vi "loadTestTime.vi"() -> ()   [LabVIEW 2012]
uses:
  <vilib>/addons/database/Connection.llb/DB Tools Open Connec (Path).vi
  <vilib>/addons/database/Connection.llb/Conn Execute.vi
  <vilib>/addons/database/Recordset.llb/Rec Destroy - Connection.vi
  <vilib>/addons/database/Recordset.llb/Rec Fetch Recordset Data (R).vi
  <vilib>/addons/database/Recordset.llb/Rec Fetch Integer Data (R).vi
  <vilib>/addons/database/_DB Variant To Data/Database Variant To Data.xnode
  <vilib>/addons/database/NI_Database_API.lvlib
panel:
  out "error out":errorcluster
  in  "Cluster":T1
  out "output cluster":T1
  out "concatenated string 3":string
  out "appended array":string[](array[string])
  out "concatenated string":string
  out "Second":dbl
  out "concatenated string 2":string
  out "TestSec":dbl
  out "Temp":i32
  out "appended array 2":i32[](array[numeric])
  out "x/y":dbl
  out "substring":string
  out "x .or. y?":bool
  out "x > y?":bool
  out "data":string
  out "error out 2":errorcluster
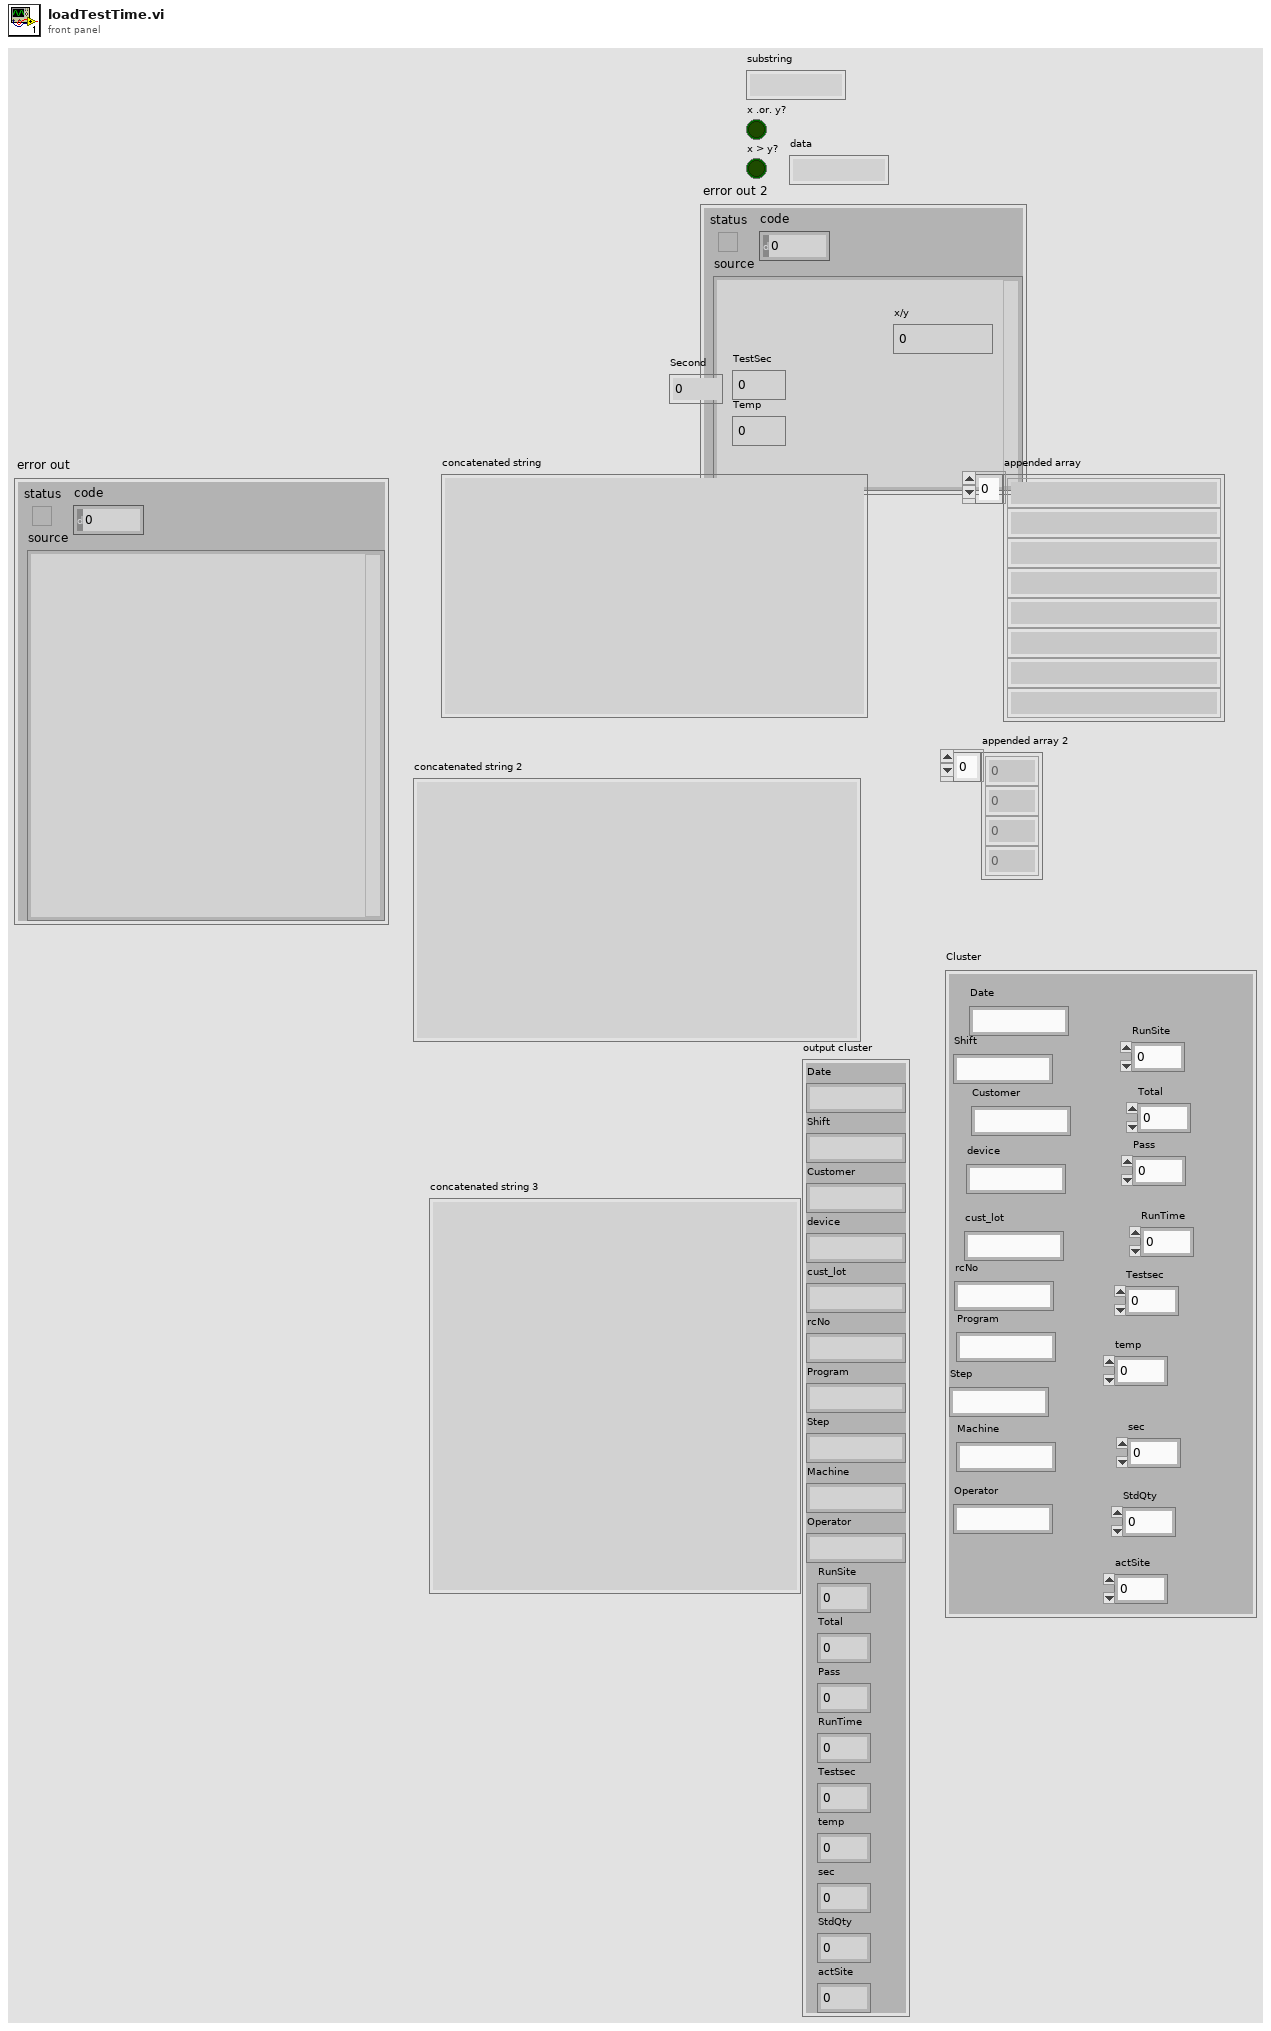
[diagram p1: front panel]
types:
  T1 = cluster{"Date":string, "Shift":string, "Customer":string, "device":string, "cust_lot":string, "rcNo":string, "Program":string, "Step":string, "Machine":string, "Operator":string, "RunSite":dbl, "Total":dbl, "Pass":dbl, "RunTime":dbl, "Testsec":dbl, "temp":dbl, "sec":dbl, "StdQty":dbl, "actSite":dbl}
  T2 = typedef "NI_Database_API.lvlib/Conn ObjectReference.ctl" = refnum<k1>
  T3 = typedef "NI_Database_API.lvlib/Rec ObjectReference.ctl" = refnum<k1>
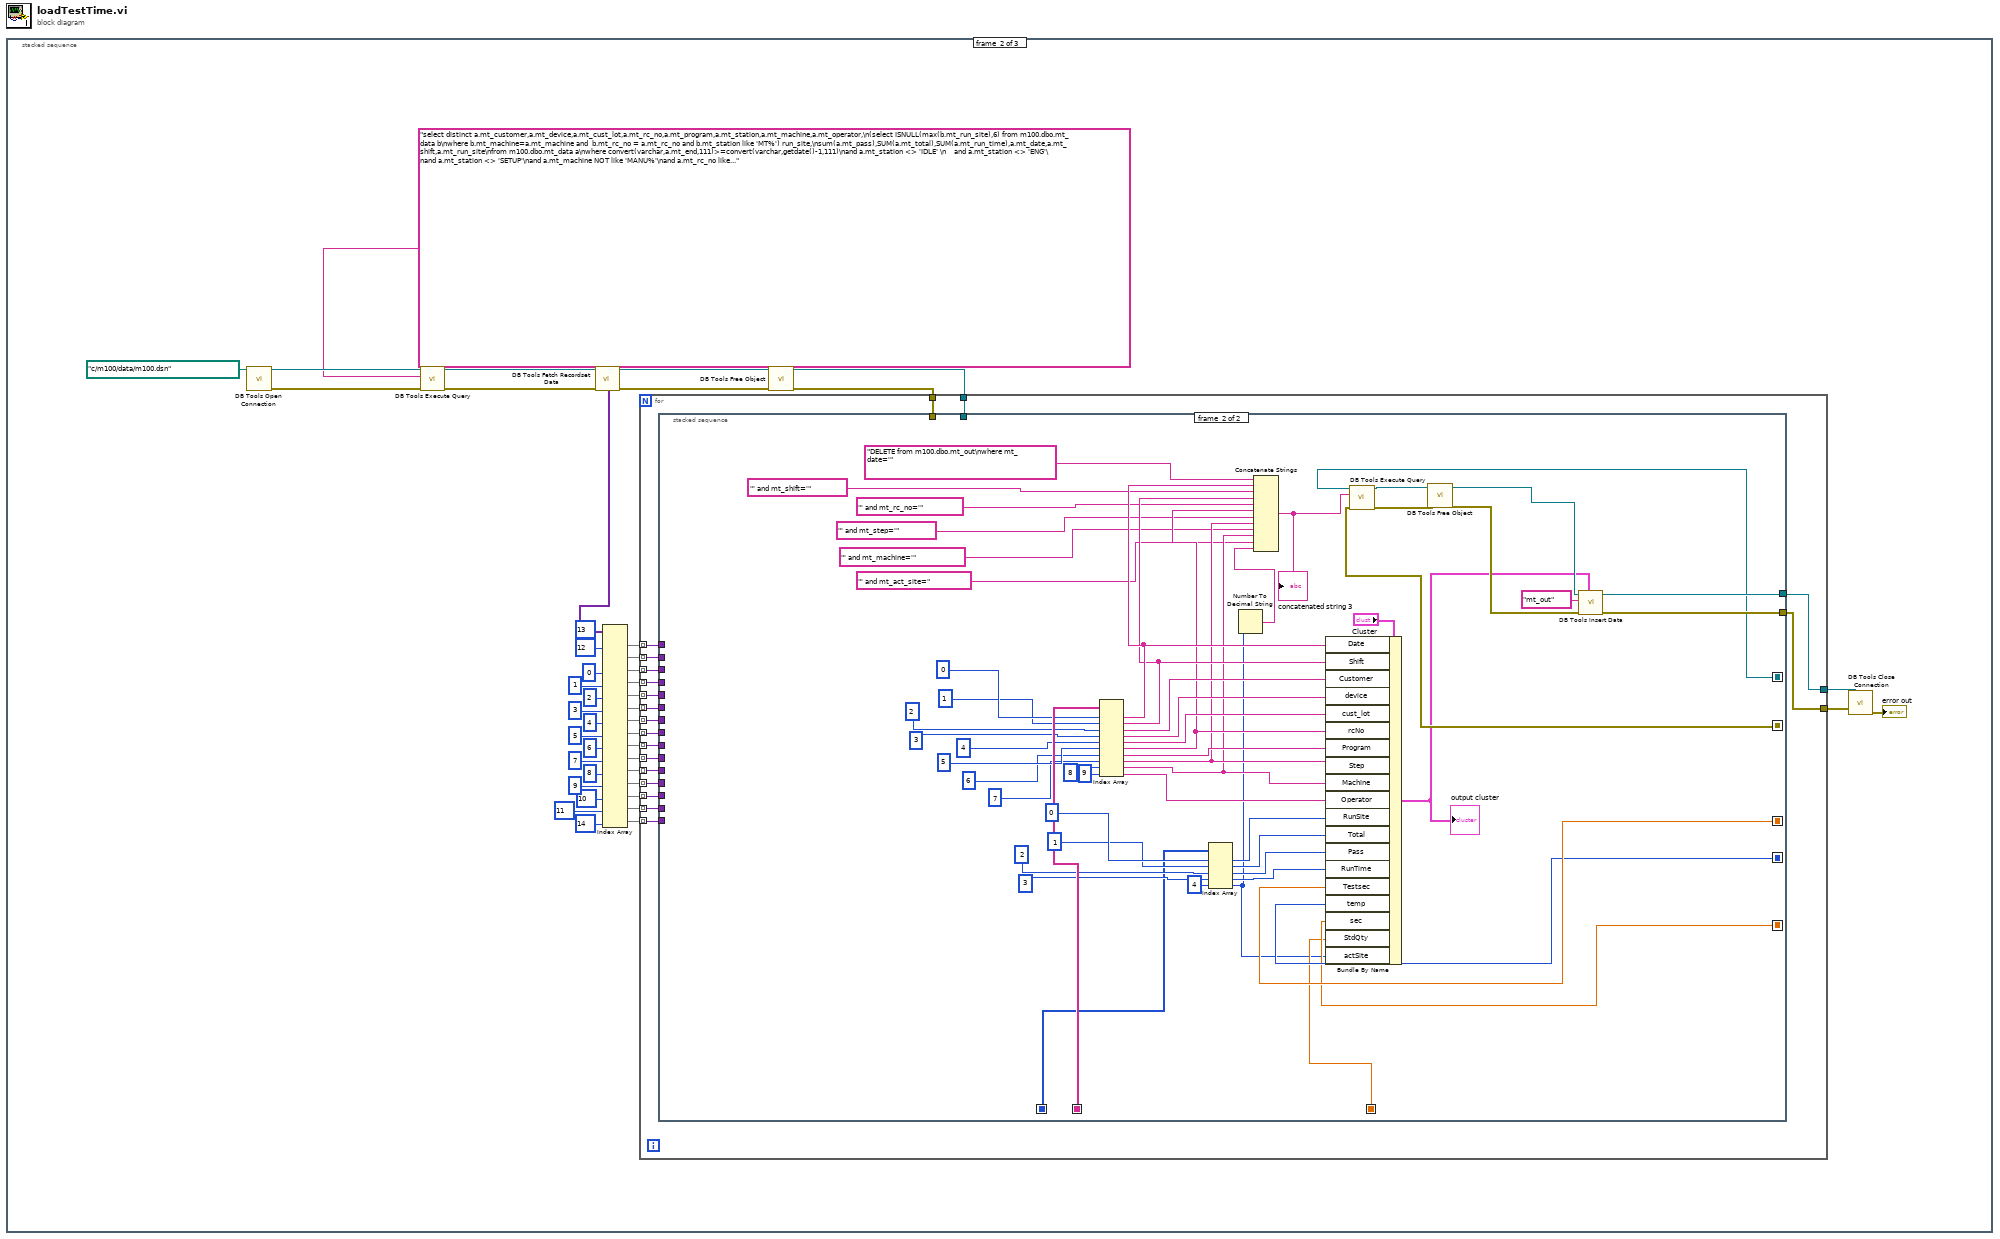
[diagram p0: block diagram]
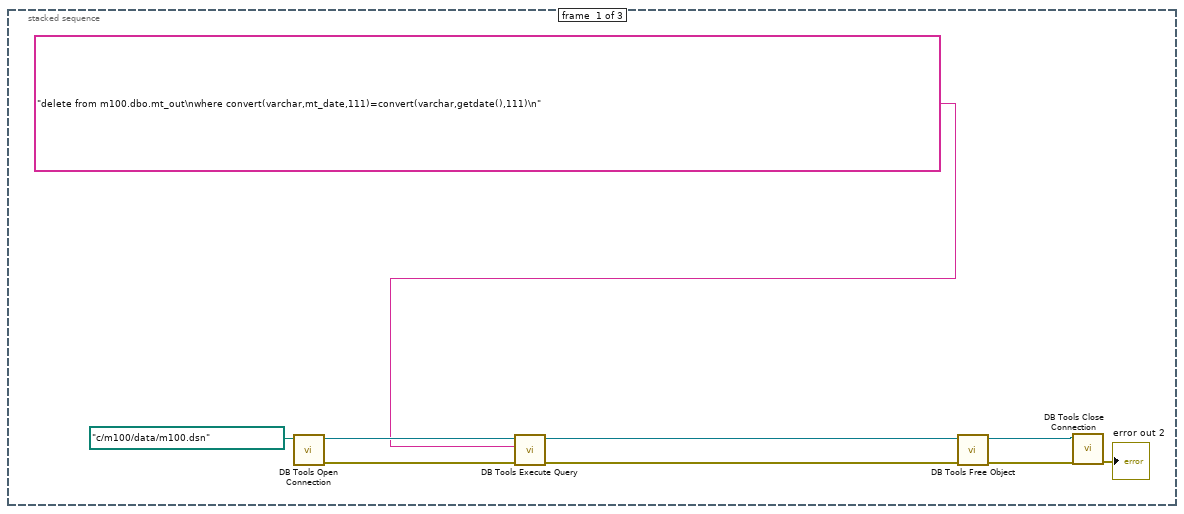
[diagram p2: hidden frame]
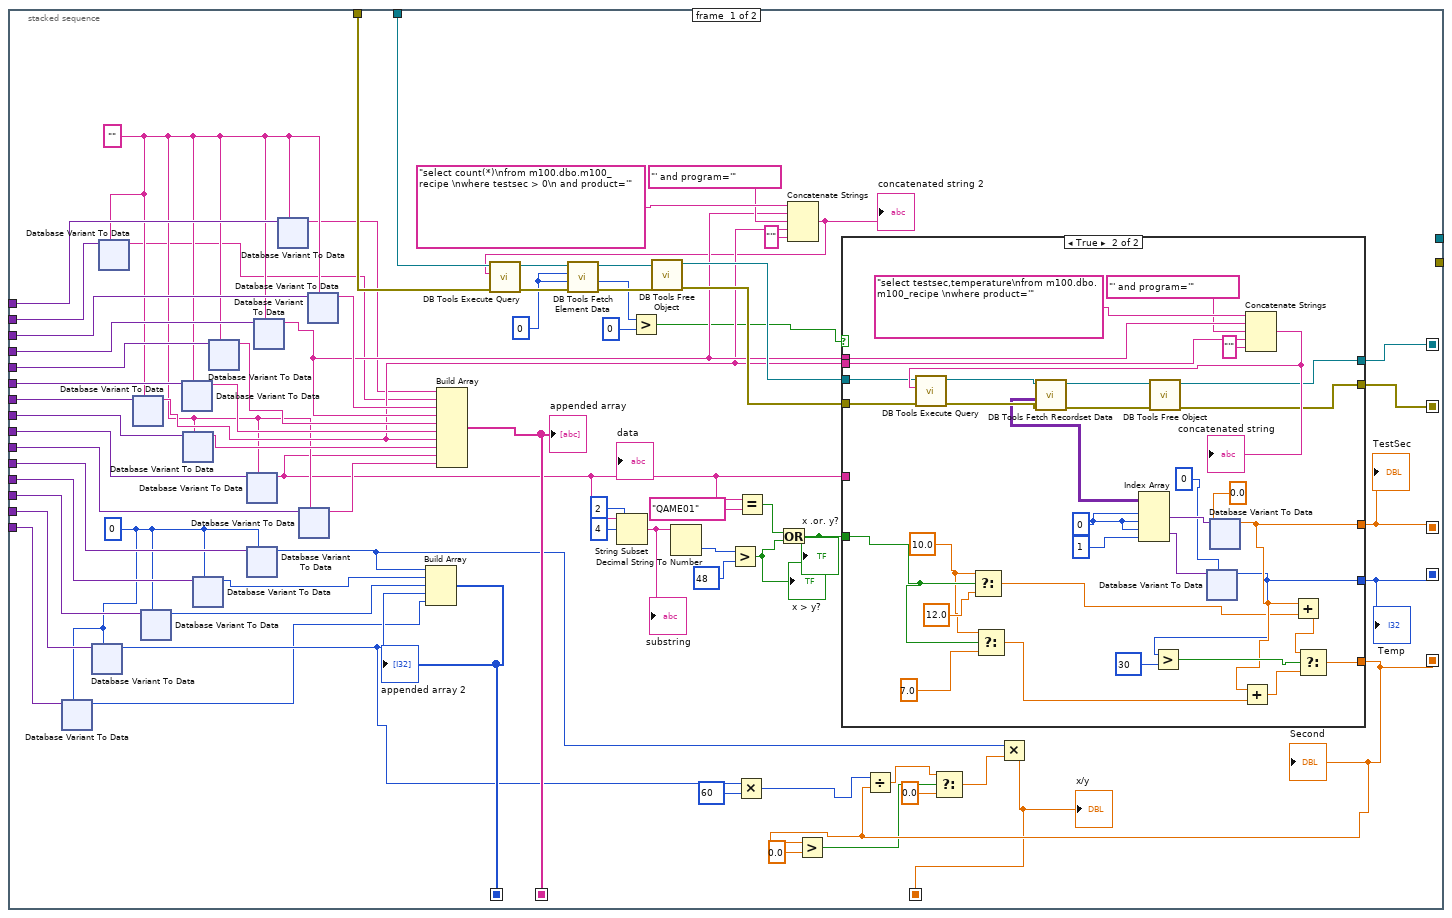
[diagram p3: hidden frame]
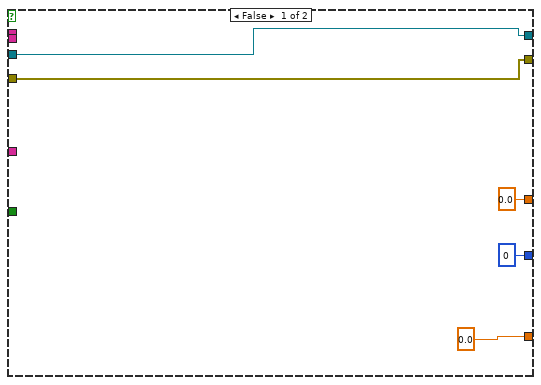
[diagram p4: hidden frame]
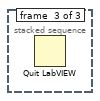
[diagram p5: hidden frame]
diagram:
  n1 = stacked-sequence {
    frame #0 {
      n2 = call-poly <vilib>:"DB Tools Open Connection.vi"("connection information"=path "c:/m100/data/m100.dsn") -> ("error out"=w8:errorcluster, "connection reference"=w9:T2)  [unwired: 7 in]
      n3 = call-poly <vilib>:"DB Tools Execute Query.vi"("error in (no error)"=w8, "SQL query"="delete from m100.dbo.mt_out\nwhere convert(varchar,mt_date,111)=convert(varchar,getdate(),111)\n", "connection reference"=w9) -> ("error out"=w4:errorcluster, "recordset reference"=w5:T3)  [unwired: 5 in]
      n4 = call-poly <vilib>:"DB Tools Free Object.vi"("error in (no error)"=w4, "recordset reference"=w5) -> ("error out"=w2:errorcluster, "connection reference"=w3:T2)  [unwired: 8 in]
      n5 = call <vilib>:"DB Tools Close Connection.vi"("error in (no error)"=w2, "connection reference"=w3) -> ("error out"=→"error out 2":errorcluster)  [unwired: 5 in]
    }
    frame #1 {
      n6 = call-poly <vilib>:"DB Tools Open Connection.vi"("connection information"=path "c:/m100/data/m100.dsn") -> ("error out"=w50:errorcluster, "connection reference"=w53:T2)  [unwired: 7 in]
      n7 = call-poly <vilib>:"DB Tools Execute Query.vi"("error in (no error)"=w50, "SQL query"="select distinct a.mt_customer,a.mt_device,a.mt_cust_lot,a.mt_rc_no,a.mt_program,a.mt_station,a.mt_machine,a.mt_operator,\n(select ISNULL(max(b.mt_run_site),6) from m100.dbo.mt_data b\nwhere b.mt_machine=a.mt_machine and  b.mt_rc_no = a.mt_rc_no and b.mt_station like 'MT%') run_site,\nsum(a.mt_pass),SUM(a.mt_total),SUM(a.mt_run_time),a.mt_date,a.mt_shift,a.mt_run_site\nfrom m100.dbo.mt_data a\nwhere convert(varchar,a.mt_end,111)>=convert(varchar,getdate()-1,111)\nand a.mt_station <> 'IDLE' \n    and a.mt_station <> 'ENG'\nand a.mt_station <> 'SETUP'\nand a.mt_machine NOT like 'MANU%'\nand a.mt_rc_no like 'A%'\ngroup by  mt_date,mt_shift,mt_customer,mt_device,mt_cust_lot,mt_rc_no,mt_program,mt_station,mt_machine,mt_operator,mt_run_site", "connection reference"=w53) -> ("error out"=w49:errorcluster, "recordset reference"=w52:T3)  [unwired: 5 in]
      n8 = call-poly <vilib>:"DB Tools Fetch Recordset Data.vi"("error in (no error)"=w49, "recordset reference"=w52) -> ("error out"=w48:errorcluster, "recordset data"=w44:variant[][], "recordset reference out"=w51:T3)  [unwired: 3 in]
      n9 = Index Array(array=w44, index (col) #1=12 ("disabled index (col)"), index (col) #2=13 ("index (col)"), index (col) #3=0 ("disabled index (col)"), index (col) #4=1 ("index (col)"), index (col) #5=2 ("index (col)"), index (col) #6=3 ("index (col)"), index (col) #7=4 ("index (col)"), index (col) #8=5 ("index (col)"), index (col) #9=6 ("index (col)"), index (col) #10=7 ("index (col)"), index (col) #11=8 ("index (col)"), index (col) #12=9 ("index (col)"), index (col) #13=10 ("index (col)"), index (col) #14=11 ("index (col)"), index (col) #15=14 ("index (col)")) -> (element #1=w13:variant[], element #2=w12:variant[], element #3=w28:variant[], element #4=w29:variant[], element #5=w30:variant[], element #6=w35:variant[], element #7=w34:variant[], element #8=w33:variant[], element #9=w32:variant[], element #10=w31:variant[], element #11=w19:variant[], element #12=w18:variant[], element #13=w17:variant[], element #14=w16:variant[], element #15=w10:variant[])  [unwired: 15 in]
      n10 = call-poly <vilib>:"DB Tools Free Object.vi"("error in (no error)"=w48, "recordset reference"=w51) -> ("error out"=w26:errorcluster, "connection reference"=w27:T2)  [unwired: 8 in]
      n11 = for {
        tunnel: w35 -> [w72] mode=indexing
        tunnel: w34 -> [w71] mode=indexing
        tunnel: w33 -> [w70] mode=indexing
        tunnel: w32 -> [w69] mode=indexing
        tunnel: w31 -> [w68] mode=indexing
        tunnel: w30 -> [w67] mode=indexing
        tunnel: w29 -> [w66] mode=indexing
        tunnel: w28 -> [w65] mode=indexing
        tunnel: w27 -> [w64]
        tunnel: w26 -> [w63]
        tunnel: [w56] -> w25
        tunnel: [w55] -> w24
        tunnel: w19 -> [w62] mode=indexing
        tunnel: w18 -> [w61] mode=indexing
        tunnel: w17 -> [w60] mode=indexing
        tunnel: w16 -> [w59] mode=indexing
        tunnel: w13 -> [w58] mode=indexing
        tunnel: w12 -> [w57] mode=indexing
        tunnel: w10 -> [w54] mode=indexing
        n12 = stacked-sequence {
          seq-local: [w106 _] -> [_ w757]
          seq-local: [w107 _] -> [_ w756]
          seq-local: [w93 _] -> [_ w755]
          seq-local: [w105 _] -> [_ w761]
          seq-local: [w104 _] -> [_ w781]
          seq-local: [w87 _] -> [_ w734]
          seq-local: [w95 _] -> [_ w738]
          seq-local: [w94 _] -> [_ w737]
          tunnel: w72 -> [w144 _]
          tunnel: w71 -> [w143 _]
          tunnel: w70 -> [w142 _]
          tunnel: w69 -> [w141 _]
          tunnel: w68 -> [w140 _]
          tunnel: w67 -> [w139 _]
          tunnel: w66 -> [w138 _]
          tunnel: w65 -> [w137 _]
          tunnel: w64 -> [w131 _]
          tunnel: w63 -> [w130 _]
          tunnel: w62 -> [w113 _]
          tunnel: w61 -> [w112 _]
          tunnel: w60 -> [w111 _]
          tunnel: w59 -> [w110 _]
          tunnel: w58 -> [w103 _]
          tunnel: w57 -> [w102 _]
          tunnel: [_ w754] -> w56
          tunnel: [_ w753] -> w55
          tunnel: w54 -> [w75 _]
          frame #0 {
            w74 = 0
            w117 = 0
            w101 = ""
            n13 = xnode "Database Variant To Data"("database variant"=w75, "type"=w74) -> ("data"=w73:i32)  [unwired: 1 in, 1 out]
            n14 = xnode "Database Variant To Data"("database variant"=w110, "type"=w74) -> ("data"=w98:i32)  [unwired: 1 in, 1 out]
            n15 = xnode "Database Variant To Data"("database variant"=w102, "type"=w101) -> ("data"=w99:string)  [unwired: 1 in, 1 out]
            n16 = xnode "Database Variant To Data"("database variant"=w143, "type"=w101) -> ("data"=w119:string)  [unwired: 1 in, 1 out]
            n17 = xnode "Database Variant To Data"("database variant"=w111, "type"=w74) -> ("data"=w108:i32)  [unwired: 1 in, 1 out]
            n18 = xnode "Database Variant To Data"("database variant"=w144, "type"=w101) -> ("data"=w134:string)  [unwired: 1 in, 1 out]
            n19 = xnode "Database Variant To Data"("database variant"=w142, "type"=w101) -> ("data"=w133:string)  [unwired: 1 in, 1 out]
            n20 = xnode "Database Variant To Data"("database variant"=w112, "type"=w74) -> ("data"=w109:i32)  [unwired: 1 in, 1 out]
            n21 = xnode "Database Variant To Data"("database variant"=w139, "type"=w101) -> ("data"=w135:string)  [unwired: 1 in, 1 out]
            n22 = xnode "Database Variant To Data"("database variant"=w141, "type"=w101) -> ("data"=w81:string)  [unwired: 1 in, 1 out]
            "data" <- w81
            n23 = xnode "Database Variant To Data"("database variant"=w113, "type"=w74) -> ("data"=w86:i32)  [unwired: 1 in, 1 out]
            n24 = xnode "Database Variant To Data"("database variant"=w138, "type"=w101) -> ("data"=w120:string)  [unwired: 1 in, 1 out]
            n25 = xnode "Database Variant To Data"("database variant"=w103, "type"=w101) -> ("data"=w100:string)  [unwired: 1 in, 1 out]
            n26 = xnode "Database Variant To Data"("database variant"=w140, "type"=w101) -> ("data"=w132:string)  [unwired: 1 in, 1 out]
            n27 = xnode "Database Variant To Data"("database variant"=w137, "type"=w101) -> ("data"=w136:string)  [unwired: 1 in, 1 out]
            n28 = Build Array(w86, w109, w108, w98, w73) -> (w105:i32[])
            "appended array 2" <- w105
            n29 = Build Array(w100, w99, w136, w120, w135, w134, w119, w133, w81, w132) -> (w104:string[])
            "appended array" <- w104
            n30 = String Subset(string=w81, offset (0)=4, length (rest)=2 ("length (rest)")) -> (substring=w84:string)
            "substring" <- w84
            n31 = Decimal String To Number(string=w84) -> (number=w83:i32)  [unwired: 2 in, 1 out]
            n32 = Greater?(x=w83, y=48) -> (0:w78:bool)
            "x > y?" <- w78
            n33 = Multiply(x=w98, y=60) -> (x*y=w96:i32)
            n34 = Equal?(x=w81, y="QAME01") -> (x = y?=w79:bool)
            n35 = Or(x=w79, y=w78) -> (x .or. y?=w77:bool)
            "x .or. y?" <- w77
            n36 = Concatenate Strings("select count(*)\nfrom m100.dbo.m100_recipe \nwhere testsec > 0\n and product='" ("SQL query"), w120, "' and program='" ("string"), w119, "'" ("string")) -> (w118:string)
            "concatenated string 2" <- w118
            n37 = call-poly <vilib>:"DB Tools Execute Query.vi"("error in (no error)"=w130, "SQL query"=w118, "connection reference"=w131) -> ("error out"=w128:errorcluster, "recordset reference"=w129:T3)  [unwired: 5 in]
            n38 = call-poly <vilib>:"DB Tools Fetch Element Data.vi"("error in (no error)"=w128, "type"=w117, "column index"=w117, "recordset reference"=w129) -> ("error out"=w126:errorcluster, "data"=w116:i32, "recordset reference out"=w127:T3)  [unwired: 3 in]
            n39 = Greater?(x=w116, y=0) -> (0:w114:bool)
            n40 = call-poly <vilib>:"DB Tools Free Object.vi"("error in (no error)"=w126, "recordset reference"=w127) -> ("error out"=w124:errorcluster, "connection reference"=w125:T2)  [unwired: 8 in]
            n41 = case shown="True" w114 {
              tunnel: w120 -> [_ w402]
              tunnel: w119 -> [_ w400]
              tunnel: w125 -> [w373 w397]
              tunnel: w124 -> [w372 w396]
              tunnel: [w373 w395] -> w95
              tunnel: [w372 w394] -> w94
              tunnel: [0.0 w382] -> w93
              tunnel: [0.0 ("data") w381] -> w106
              tunnel: [0 ("data") w380] -> w107
              tunnel: w81 -> [_ _]
              tunnel: w77 -> [_ w379]
              frame False {
              }
              frame True {
                w376 = 10.0 ("t")
                w391 = 0 ("disabled index (col)")
                n42 = Select(t=w376, s=w379, f=12.0 ("y")) -> (s? t:f=w377:dbl)
                n43 = Select(t=w376, s=w379, f=7.0 ("y")) -> (s? t:f=w374:dbl)
                n44 = Concatenate Strings("select testsec,temperature\nfrom m100.dbo.m100_recipe \nwhere product='" ("SQL query"), w402, "' and program='" ("string"), w400, "'" ("string")) -> (w399:string)
                "concatenated string" <- w399
                n45 = call-poly <vilib>:"DB Tools Execute Query.vi"("error in (no error)"=w396, "SQL query"=w399, "connection reference"=w397) -> ("error out"=w406:errorcluster, "recordset reference"=w407:T3)  [unwired: 5 in]
                n46 = call-poly <vilib>:"DB Tools Fetch Recordset Data.vi"("error in (no error)"=w406, "recordset reference"=w407) -> ("error out"=w404:errorcluster, "recordset data"=w393:variant[][], "recordset reference out"=w405:T3)  [unwired: 3 in]
                n47 = Index Array(array=w393, index (row) #1=w391, index (col) #1=w391, index (row) #2=w391, index (col) #2=1 ("index (col)")) -> (element #1=w390:variant, element #2=w389:variant)
                n48 = call-poly <vilib>:"DB Tools Free Object.vi"("error in (no error)"=w404, "recordset reference"=w405) -> ("error out"=w394:errorcluster, "connection reference"=w395:T2)  [unwired: 8 in]
                n49 = xnode "Database Variant To Data"("database variant"=w389, "type"=0) -> ("data"=w380:i32)  [unwired: 1 in, 1 out]
                n50 = Greater?(x=w380, y=30) -> (0:w385:bool)
                n51 = xnode "Database Variant To Data"("database variant"=w390, "type"=0.0) -> ("data"=w381:dbl)  [unwired: 1 in, 1 out]
                n52 = Add(x=w381, y=w374) -> (x+y=w383:dbl)
                n53 = Add(x=w381, y=w377) -> (x+y=w384:dbl)
                n54 = Select(t=w384, s=w385, f=w383) -> (s? t:f=w382:dbl)
              }
            }
            "Second" <- w93
            "TestSec" <- w106
            "Temp" <- w107
            n55 = Greater?(x=w93, y=0.0) -> (0:w90:bool)
            n56 = Divide(x=w96, y=w93) -> (x/y=w91:dbl)
            n57 = Select(t=w91, s=w90, f=0.0) -> (s? t:f=w88:dbl)
            n58 = Multiply(x=w86, y=w88) -> (x*y=w87:dbl)
            "x/y" <- w87
          }
          frame #1 {
            n59 = Index Array(array=w781, index #1=0 ("index"), index #2=1 ("index"), index #3=2 ("index"), index #4=3 ("index"), index #5=4 ("index"), index #6=5 ("index"), index #7=6 ("index"), index #8=7 ("index"), index #9=8 ("index"), index #10=9 ("index")) -> (element #1=w751:string, element #2=w749:string, element #3=w770:string, element #4=w769:string, element #5=w768:string, element #6=w747:string, element #7=w767:string, element #8=w745:string, element #9=w743:string, element #10=w766:string)
            n60 = Index Array(array=w761, index #1=0 ("index"), index #2=1 ("index"), index #3=2 ("index"), index #4=3 ("index"), index #5=4 ("index")) -> (element #1=w741:i32, element #2=w760:i32, element #3=w759:i32, element #4=w758:i32, element #5=w728:i32)
            n61 = Number To Decimal String(number=w728) -> (decimal integer string=w740:string)  [unwired: 1 in]
            n62 = Concatenate Strings("DELETE from m100.dbo.mt_out\nwhere mt_date='", w751, "' and mt_shift='" ("string"), w749, "' and mt_rc_no='" ("string"), w747, "' and mt_step='" ("string"), w745, "' and mt_machine='" ("string"), w743, "' and mt_act_site=" ("string"), w740) -> (w739:string)
            "concatenated string 3" <- w739
            n63 = Bundle By Name(cluster="Cluster", "Date"=w751, "Shift"=w749, "Customer"=w770, "device"=w769, "cust_lot"=w768, "rcNo"=w747, "Program"=w767, "Step"=w745, "Machine"=w743, "Operator"=w766, "RunSite"=w741, "Total"=w760, "Pass"=w759, "RunTime"=w758, "Testsec"=w757, "temp"=w756, "sec"=w755, "StdQty"=w734, "actSite"=w728) -> (w732:T1)
            "output cluster" <- w732
            n64 = call-poly <vilib>:"DB Tools Execute Query.vi"("error in (no error)"=w737, "SQL query"=w739, "connection reference"=w738) -> ("error out"=w729:errorcluster, "recordset reference"=w730:T3)  [unwired: 5 in]
            n65 = call-poly <vilib>:"DB Tools Free Object.vi"("error in (no error)"=w729, "recordset reference"=w730) -> ("error out"=w735:errorcluster, "connection reference"=w736:T2)  [unwired: 8 in]
            n66 = call <vilib>:"DB Tools Insert Data.vi"("data"=w732, "error in (no error)"=w735, "table"="mt_out", "connection reference"=w736) -> ("error out"=w753:errorcluster, "connection reference out"=w754:T2)  [unwired: 6 in]
          }
        }
      }
      n67 = call <vilib>:"DB Tools Close Connection.vi"("error in (no error)"=w24, "connection reference"=w25) -> ("error out"=→"error out":errorcluster)  [unwired: 5 in]
    }
    frame #2 {
      n68 = Quit LabVIEW() -> ()  [unwired: 1 in]
    }
  }
